vi "Shot Overlay 2 (SubVI).vi"(6 "Image Out":T1, 7 "Particle Measurements (Pixels) (Particle Analysis 1)":dbl[][](array[numeric]), 8 "Particle Measurements (Real-World) (Particle Analysis 1)":dbl[][](array[numeric]), 9 "Nb Circles (Circle Detection 1)":i32) -> (1 "Shot Overlay":T1, 2 "Player Position Pixels":dbl[][](array[numeric]), 3 "Puck position pixels":dbl[][](array[numeric]))   [LabVIEW 2013]
uses:
  <vilib>/vision/Image Controls.llb/IMAQ Image.ctl
panel:
  out "error out":errorcluster
  out "Shot Overlay":T1(plugin-control)
  out "element y":dbl
  out "element x":dbl
  out "Player area overlay":T1
  out "output cluster":cluster{i32, i32, i32, i32}
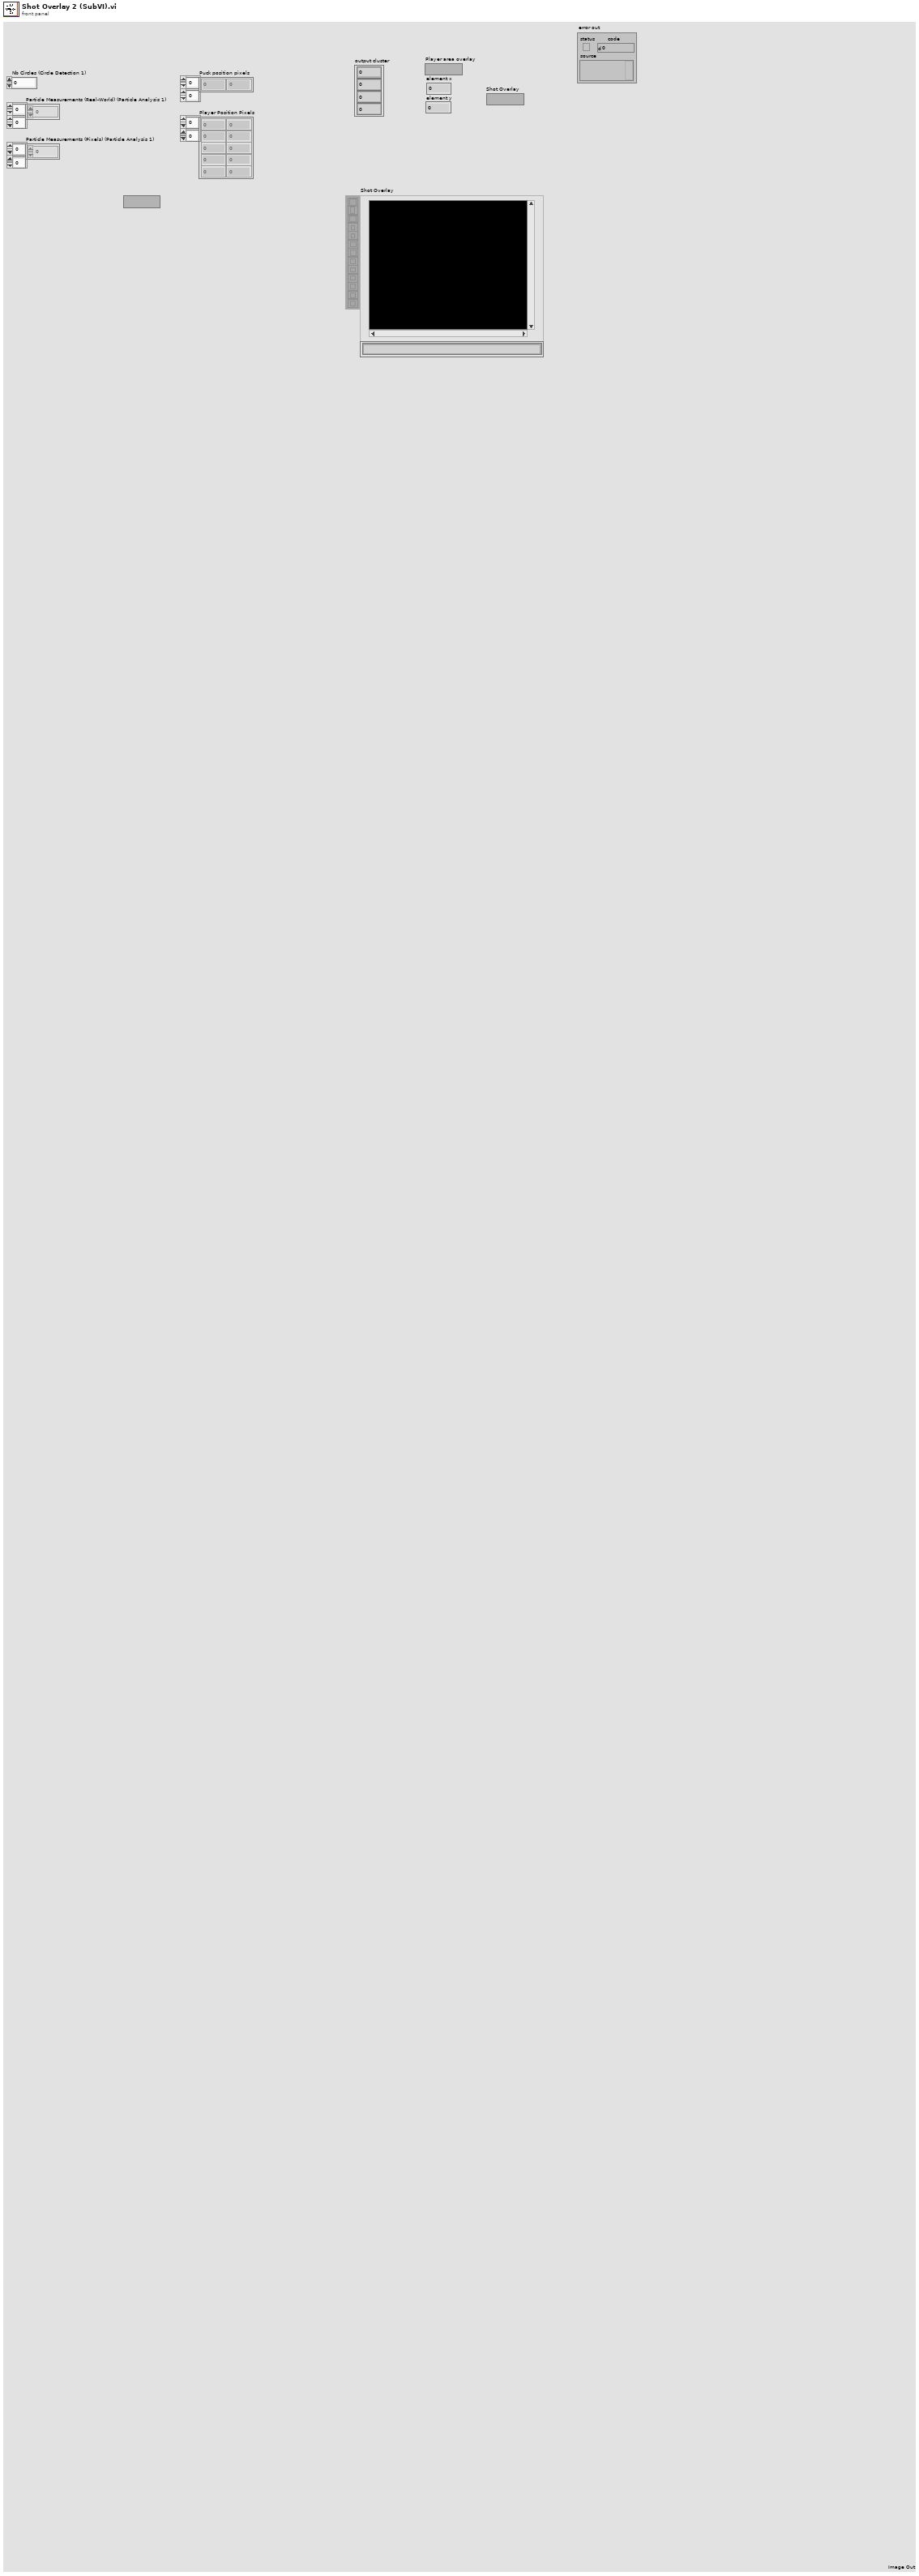
[diagram p1: front panel]
types:
  T1 = typedef "IMAQ Image.ctl" = refnum<image>
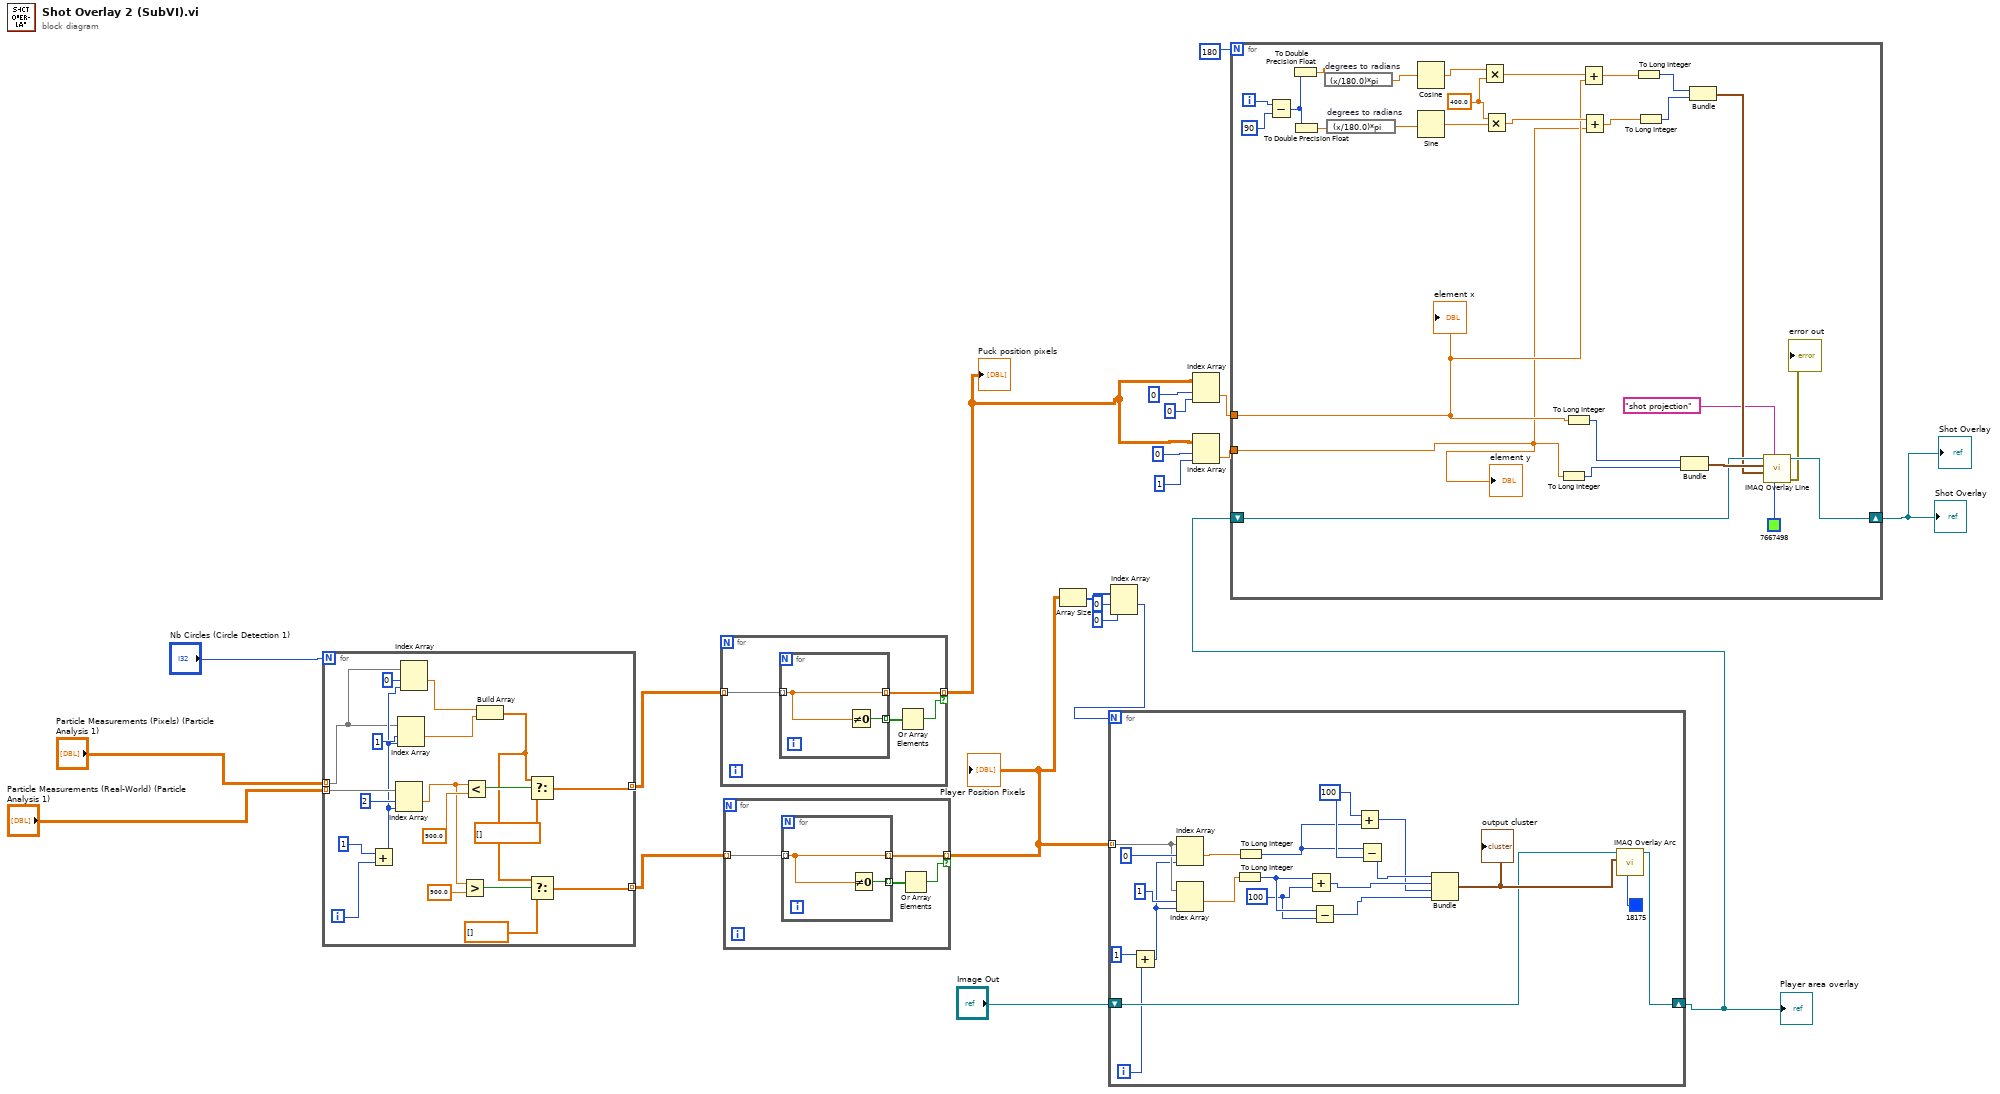
[diagram p0: block diagram]
diagram:
  n1 = for {
    N: "Nb Circles (Circle Detection 1)" -> [_]
    tunnel: "Particle Measurements (Real-World) (Particle Analysis 1)" -> [w34] mode=indexing
    tunnel: [w36] -> w18 mode=indexing
    tunnel: [w23] -> w19 mode=indexing
    tunnel: "Particle Measurements (Pixels) (Particle Analysis 1)" -> [w22] mode=indexing
    i -> [w40]
    n2 = Add(x=1, y=w40) -> (x+y=w32:i32)
    n3 = Index Array(array=w34, index #1=2 ("index"), index #2=w32) -> (element #1=w27:dbl)  [unwired: 1 out]
    n4 = Index Array(array=w22, index #1=1 ("index"), index #2=w32) -> (element #1=w30:dbl)  [unwired: 1 out]
    n5 = Index Array(array=w22, index #1=0 ("index"), index #2=w32) -> (element #1=w31:dbl)  [unwired: 1 out]
    n6 = Greater?(x=w27, y=900.0) -> (0:w26:bool)
    n7 = Less?(x=w27, y=900.0) -> (x < y?=w37:bool)
    n8 = Build Array(w31, w30) -> (w25:dbl[])
    n9 = Select(t=w25, s=w37, f=dbl[] []) -> (s? t:f=w36:dbl[])
    n10 = Select(t=w25, s=w26, f=dbl[] []) -> (s? t:f=w23:dbl[])
  }
  n11 = for {
    tunnel: w18 -> [w45] mode=indexing
    tunnel: [w43] -> w6 mode=indexing if=w42
    n12 = for {
      tunnel: w45 -> [w46] mode=indexing
      tunnel: [w47] -> w44 mode=indexing
      tunnel: [w46] -> w43 mode=indexing
      n13 = Not Equal To 0?(x=w46) -> (x != 0?=w47:bool)
    }
    n14 = Or Array Elements(Boolean array=w44) -> (logical OR=w42:bool)
  }
  "Puck position pixels" <- w6
  n15 = for {
    tunnel: w19 -> [w51] mode=indexing
    tunnel: [w49] -> w12 mode=indexing if=w48
    n16 = for {
      tunnel: w51 -> [w52] mode=indexing
      tunnel: [w53] -> w50 mode=indexing
      tunnel: [w52] -> w49 mode=indexing
      n17 = Not Equal To 0?(x=w52) -> (x != 0?=w53:bool)
    }
    n18 = Or Array Elements(Boolean array=w50) -> (logical OR=w48:bool)
  }
  "Player Position Pixels" <- w12
  n19 = Array Size(array=w12) -> (size(s)=w15:i32[])
  n20 = Index Array(array=w15, index #1=0 ("index"), index #2=0 ("index")) -> (element #1=w11:i32)  [unwired: 1 out]
  n21 = for {
    N: w11 -> [_]
    tunnel: w12 -> [w57] mode=indexing
    shift-right: [w61] -> w10
    shift-left: "Image Out" -> [w62]
    i -> [w59]
    w69 = 100 ("y")
    w73 = 100 ("x")
    n22 = Add(x=1, y=w59) -> (x+y=w55:i32)
    n23 = Index Array(array=w57, index #1=0 ("index"), index #2=w55) -> (element #1=w72:dbl)  [unwired: 1 out]
    n24 = Index Array(array=w57, index #1=1 ("index"), index #2=w55) -> (element #1=w54:dbl)  [unwired: 1 out]
    n25 = To Long Integer(number=w54) -> (32bit integer=w70:i32)
    n26 = To Long Integer(number=w72) -> (32bit integer=w71:i32)
    n27 = Add(x=w70, y=w69) -> (x+y=w67:i32)
    n28 = Subtract(x=w70, y=w69) -> (x-y=w65:i32)
    n29 = Add(x=w73, y=w71) -> (x+y=w66:i32)
    n30 = Subtract(x=w71, y=w73) -> (x-y=w68:i32)
    n31 = Bundle(w68, w67, w66, w65) -> (w63:cluster{i32, i32, i32, i32})  [unwired: 1 in]
    "output cluster" <- w63
    n32 = call "IMAQ Overlay Arc"("Color"=u32 18175, "Bounding Rectangle"=w63, "Image"=w62) -> ("Image Out"=w61:T1)  [unwired: 7 in, 1 out]
  }
  "Player area overlay" <- w10
  n33 = Index Array(array=w6, index (row)=0, index (col)=0 ("disabled index (col)")) -> (element=w5:dbl)
  n34 = Index Array(array=w6, index (row)=0 ("index"), index (col)=1 ("disabled index (col)")) -> (element=w2:dbl)
  n35 = for {
    N: 180 ("Numeric") -> [_]
    shift-right: [w96] -> w9
    shift-left: w10 -> [w97]
    tunnel: w5 -> [w85]
    tunnel: w2 -> [w84]
    i -> [w80]
    w93 = 400.0 ("y")
    n36 = Subtract(x=w80, y=90) -> (x-y=w76:i32)
    n37 = To Double Precision Float(number=w76) -> (double precision float=w77:dbl)
    n38 = To Double Precision Float(number=w76) -> (double precision float=w75:dbl)
    n39 = expression code="(x/180.0)*pi" "degrees to radians"(w77) -> (w78:dbl)
    n40 = expression code="(x/180.0)*pi" "degrees to radians"(w75) -> (w87:dbl)
    n41 = Cosine(x=w78) -> (cos(x)=w95:dbl)
    n42 = Sine(x=w87) -> (sin(x)=w94:dbl)
    n43 = Multiply(x=w95, y=w93) -> (x*y=w74:dbl)
    n44 = Multiply(x=w93, y=w94) -> (x*y=w91:dbl)
    n45 = To Long Integer(number=w84) -> (32bit integer=w99:i32)
    n46 = To Long Integer(number=w85) -> (32bit integer=w100:i32)
    n47 = Add(x=w74, y=w85) -> (x+y=w92:dbl)
    n48 = Add(x=w91, y=w84) -> (x+y=w90:dbl)
    n49 = To Long Integer(number=w92) -> (32bit integer=w89:i32)
    n50 = To Long Integer(number=w90) -> (32bit integer=w88:i32)
    n51 = Bundle(w100, w99) -> (w98:cluster{i32, i32})  [unwired: 1 in]
    n52 = Bundle(w89, w88) -> (w83:cluster{i32, i32})  [unwired: 1 in]
    n53 = call "IMAQ Overlay Line"("Color"=u32 7667498, "Group"="shot projection", "End Point"=w83, "Start Point"=w98, "Image"=w97) -> ("error out"=→"error out":errorcluster, "Image Out"=w96:T1)  [unwired: 5 in]
    "element x" <- w85
    "element y" <- w84
  }
  "Shot Overlay" <- w9
  "Shot Overlay" <- w9
